vi "Queue Nested.vi"(8 "Alias":string, 9 "Priority?":bool, 10 "Msg Strategy":refnum<class "Msg Strategy.lvclass">, 11 "Base Queue jettl in":refnum<class "Base Queue jettl.lvclass">) -> (3 "Base Queue jettl out":refnum<class "Base Queue jettl.lvclass">)   [LabVIEW 2021, in "jettl.lvlib" / "Base Queue jettl.lvlib" / "Base Queue jettl.lvclass"]
uses:
  Base Queue jettl.lvclass
  Queue Mailbox/Queue Mailbox.lvlib
  C:/git/jettl/src/jettl/jettl/jettl.lvclass
  C:/git/jettl/src/jettl Msg Merge Error/Merge Error/Merge Error.lvclass
  C:/git/jettl/src/jettl/Queue jettl/Queue jettl.lvclass
  C:/git/jettl/src/jettl Msg Event Create/Event Create/Event Create.lvclass
  C:/git/jettl/src/jettl Msg Override Error/Override Error/Override Error.lvclass
  C:/git/jettl/src/jettl Msg Queue Create/Queue Create/Queue Create.lvclass
  C:/git/jettl/src/jettl Msg Setup/Setup/Setup.lvclass
  C:/git/jettl/src/jettl Msg Teardown/Teardown/Teardown.lvclass
  C:/git/jettl/src/jettl/jettl Msg Event Last Ack/Event Last Ack/Event Last Ack.lvclass
  C:/git/jettl/src/jettl/jettl Msg Queue Last Ack/Queue Last Ack/Queue Last Ack.lvclass
  C:/git/jettl/src/jettl/Base Queue jettl/Base Queue jettl/Base Queue jettl.lvclass
  Msg Strategy/Msg Strategy.lvclass
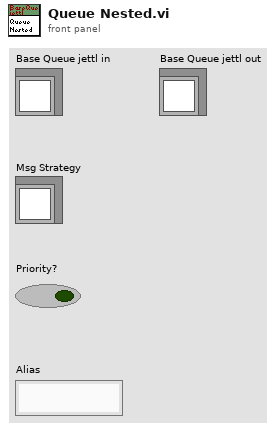
[diagram p1: front panel]
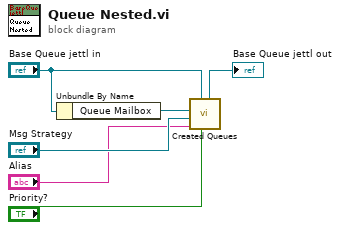
[diagram p0: block diagram]
diagram:
  n1 = Unbundle By Name("Base Queue jettl in") -> ("Queue Mailbox"=w6:refnum<data-value>)
  n2 = call "Created Queues.vi"("Created Queue Alias"="Priority?", "jettl in"="Base Queue jettl in", "Priority?"="Alias", "Msg Strategy"="Msg Strategy", "Queue Mailbox"=w6) -> ("jettl out"=→"Base Queue jettl out":refnum<class "Base Queue jettl.lvclass">)  [unwired: 6 in]
